vi "Get Setting - Error_Window_Behaviour.vi"(8 "Error In":errorcluster) -> (0 "Error Out":errorcluster, 3 "Error_Window_Behaviour":T1)   [LabVIEW 2023, in "Error Manager.lvlib" / "Settings.lvclass"]
uses:
  Settings.lvclass
  Window_Behaviour (enum).ctl
  Settings.lvclass/Settings.ctl
  Settings (class variable).vi
panel:
  # "Input\nInputs to the VI"
  # "Development\nControls or indicators that are useful for development or testing, but which are not outputs of the VI."
  # "Output\nOutputs of the VI"
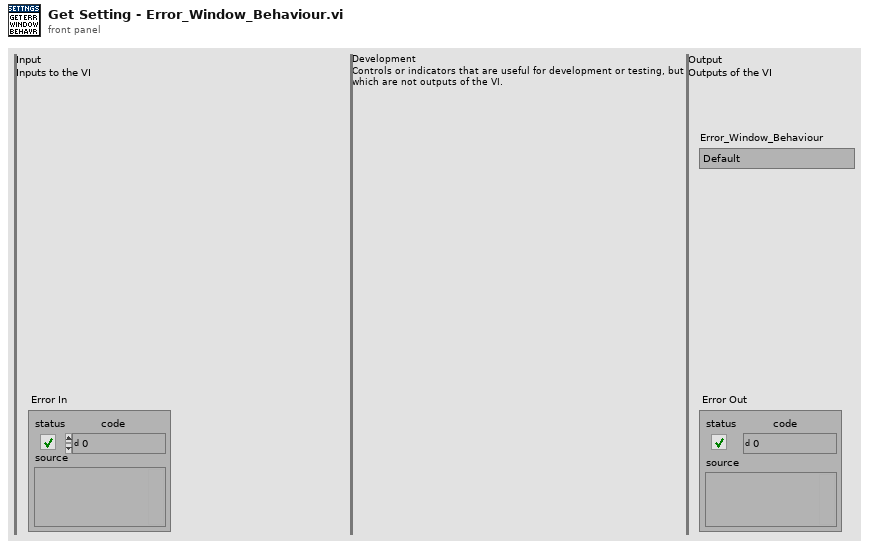
[diagram p1: front panel]
types:
  T1 = typedef "Error Manager.lvlib/Settings.lvclass/Window_Behaviour (enum).ctl" = enum16{"Default", "Floating", "Modal"}
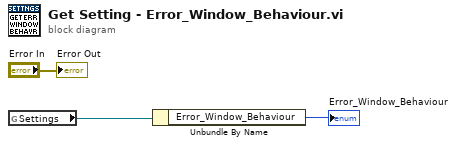
[diagram p0: block diagram]
diagram:
  n1 = global read "Settings (class variable).vi" "Settings"() -> (w1:refnum<class "Settings.lvclass">)
  n2 = Unbundle By Name(w1) -> ("Error_Window_Behaviour"=→"Error_Window_Behaviour":T1)
  "Error Out" <- "Error In"
